vi "binarize image.vi"(8 "error in (no error)":errorcluster, 11 "Thorcam in":refnum<class "Thorcam.lvclass">) -> (0 "error out":errorcluster, 3 "Thorcam out":refnum<class "Thorcam.lvclass">)   [LabVIEW 2012, in "Thorcam.lvclass"]
uses:
  Thorcam.lvclass
  Thorcam.lvclass/Thorcam.ctl
  <vilib>/vision/NI_Vision_Development_Module.lvlib
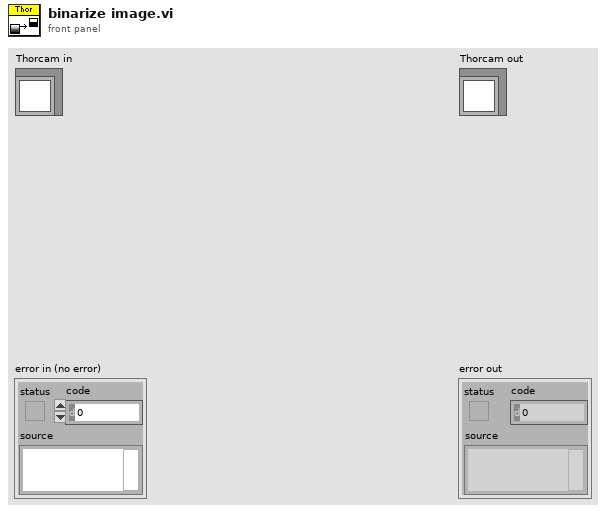
[diagram p1: front panel]
types:
  T1 = cluster{"Lower value":sgl, "Upper value":sgl, "Replace Value":sgl, "Keep/Replace Value (Replace)":bool}[]
  T2 = typedef "IMAQ Image.ctl" = refnum<image>
  T3 = cluster{"Lower value":sgl, "Upper value":sgl, "Replace Value":sgl, "Keep/Replace Value (Replace)":bool}
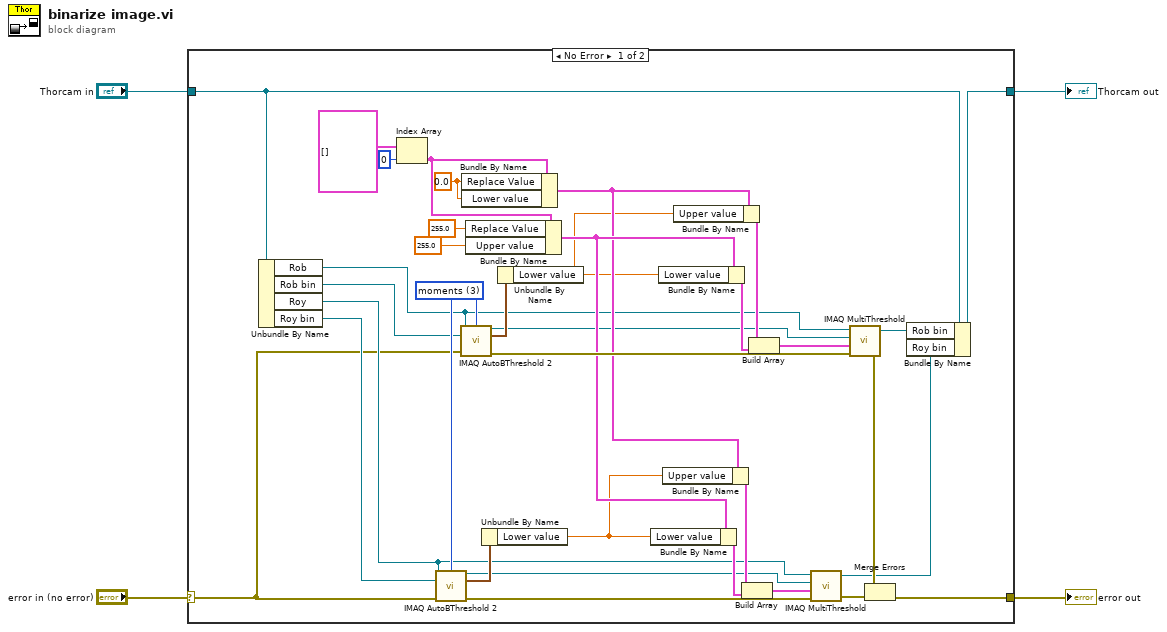
[diagram p0: block diagram]
diagram:
  n1 = case shown="No Error" "error in (no error)" {
    selector: "error in (no error)" -> [w10 w41]
    tunnel: [w9 w41] -> w3
    tunnel: [w7 w40] -> w1
    tunnel: "Thorcam in" -> [w8 w40]
    frame No Error {
      w19 = 3 items=["clustering", "entropy", "metric", "moments", "inter-class variance"] ("Method (clustering)")
      w33 = sgl 0.0 ("Replace Value")
      n2 = Unbundle By Name(w8) -> ("Rob"=w14:T2, "Rob bin"=w13:T2, "Roy"=w12:T2, "Roy bin"=w11:T2)
      n3 = Index Array(array=T1 [] ("Threshold Data"), index=0) -> (element=w34:T3)
      n4 = call "IMAQ AutoBThreshold 2"("Image Src"=w12, "Method (clustering)"=w19, "Image Dst"=w11, "error in (no error)"=w10) -> ("Image Dst Out"=w21:T2, "Threshold Range Out"=w26:cluster{"Lower value":sgl, "Upper value":sgl}, "error out"=w28:errorcluster)  [unwired: 9 in]
      n5 = call "IMAQ AutoBThreshold 2"("Image Src"=w14, "Method (clustering)"=w19, "Image Dst"=w13, "error in (no error)"=w10) -> ("Image Dst Out"=w20:T2, "Threshold Range Out"=w37:cluster{"Lower value":sgl, "Upper value":sgl}, "error out"=w36:errorcluster)  [unwired: 9 in]
      n6 = Bundle By Name(cluster=w34, "Replace Value"=w33, "Lower value"=w33) -> (w24:T3)
      n7 = Bundle By Name(cluster=w34, "Replace Value"=sgl 255.0, "Upper value"=sgl 255.0) -> (w25:T3)
      n8 = Unbundle By Name(w26) -> ("Lower value"=w16:sgl)
      n9 = Unbundle By Name(w37) -> ("Lower value"=w15:sgl)
      n10 = Bundle By Name(cluster=w25, "Lower value"=w16) -> (w22:T3)
      n11 = Bundle By Name(cluster=w25, "Lower value"=w15) -> (w30:T3)
      n12 = Bundle By Name(cluster=w24, "Upper value"=w16) -> (w23:T3)
      n13 = Bundle By Name(cluster=w24, "Upper value"=w15) -> (w31:T3)
      n14 = Build Array(w23, w22) -> (w27:T1)
      n15 = Build Array(w31, w30) -> (w29:T1)
      n16 = call "IMAQ MultiThreshold"("error in (no error)"=w28, "Threshold Data"=w27, "Image Dst"=w21, "Image Src"=w12) -> ("error out"=w18:errorcluster, "Image Dst Out"=w5:T2)  [unwired: 1 in]
      n17 = call "IMAQ MultiThreshold"("error in (no error)"=w36, "Threshold Data"=w29, "Image Dst"=w20, "Image Src"=w14) -> ("error out"=w17:errorcluster, "Image Dst Out"=w6:T2)  [unwired: 1 in]
      n18 = Merge Errors(w17, w18) -> (w9:errorcluster)
      n19 = Bundle By Name(cluster=w8, "Rob bin"=w6, "Roy bin"=w5) -> (w7:refnum<class "Thorcam.lvclass">)
    }
    frame Error {
    }
  }
  "error out" <- w3
  "Thorcam out" <- w1
